vi "Error Dialog.vi"(8 "error in (no error)":errorcluster) -> (0 "error out":errorcluster)   [LabVIEW 2016, in "System.lvlib"]
uses:
  System.lvlib
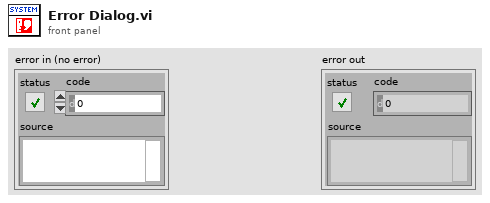
[diagram p1: front panel]
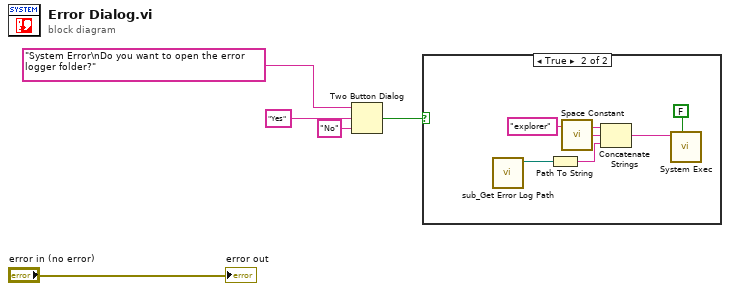
[diagram p0: block diagram]
diagram:
  n1 = Two Button Dialog(message="System Error\nDo you want to open the error logger folder?", 1:"No" ("F button name (\"Cancel\")"), 2:"Yes" ("T button name (\"OK\")")) -> (T button?=w2:bool)
  n2 = case shown="True" w2 {
    frame False {
    }
    frame True {
      n3 = call "sub_Get Error Log Path.vi"() -> ("Path"=w6:path)  [unwired: 10 in, 1 out]
      n4 = Path To String(path=w6) -> (string=w9:string)
      n5 = call <vilib>:"Space Constant.vi"() -> ("String"=w8:string)
      n6 = Concatenate Strings("explorer" ("string"), w8, w9) -> (w10:string)
      n7 = call <vilib>:"System Exec.vi"("wait until completion? (T)"=FALSE, "command line"=w10) -> ()  [unwired: 6 in, 4 out]
    }
  }
  "error out" <- "error in (no error)"
